vi "sv_Convert Units SRS.vi"(5 "desired units":i32(ring) items=["no change"=-1, "m/s^2"=0, "mm/s^2"=2, "micron/s^2"=3, "in/s^2"=1, "mil/s^2"=5], 6 "error in (no error)":errorcluster, 7 "channel info":T1={"sensor sensitivity"=1000.0, "engineering units"=1, "dB reference"=1.0, "custom label"="EU", "weighting filter"=0, "pregain"=0.0} {"pregain" format="%.2f"; "weighting filter" items=["Linear", "A-weighting", "B-weighting", "C-weighting", "ITU-R 468-4", "Dolby", "CCITT", "C-message", "Wb", "Wc", "Wd", "We", "Wf", "Wh", "Wj", "Wk", "Wm", "AES17 20 kHz lowpass", "AES17 40 kHz lowpass", "AES17 20 kHz highpass", "AES17 40 kHz highpass"]; "dB reference" format="%^.1e"; "engineering units" items=["custom..."=0, "V"=1, "A"=21, "C"=30, "pC"=31, "s"=32, "-"=29, "Pa"=2, "N"=20, "g"=3, "m/s^2"=4, "m/s"=5, "m"=6, "mm/s"=12, "mm"=13, "micron/s"=14, "micron"=15, "in/s^2"=7, "in/s"=8, "in"=9, "mil/s"=10, "mil"=11, "rad/s^2"=16, "rad/s"=17, "rad"=18, "deg/s^2"=26, "deg/s"=27, "deg"=28, "RPM"=22, "cycle/s^2"=23, "Hz"=24, "cycle"=25, "strain"=19]; "sensor sensitivity" format="%#_5f"}) -> (0 "error out":errorcluster, 1 "scale factor":dbl, 4 "unit label":string)   [LabVIEW 2017, in "SoundVib_Transient.lvlib"]
uses:
  <vilib>/addons/Sound and Vibration/svt_Transients/SoundVib_Transient.lvlib
  <vilib>/addons/_NISVFA/_Shared subVIs/Controls/svc_Channel Info.ctl
  <vilib>/addons/_NISVFA/_Shared subVIs/Controls/svc_Engineering Units Text Ring.ctl
  <vilib>/addons/_NISVFA/_Shared subVIs/Controls/svc_Weighting Filter Text Ring.ctl
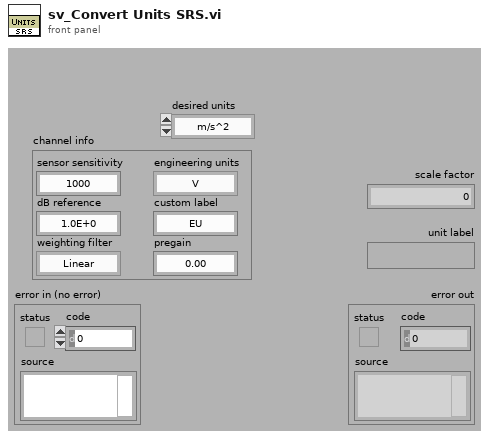
[diagram p1: front panel]
types:
  T1 = typedef "svc_Channel Info.ctl" = cluster{"sensor sensitivity":dbl, "engineering units":T2, "dB reference":dbl, "custom label":string, "weighting filter":T3, "pregain":dbl}
  T2 = typedef "svc_Engineering Units Text Ring.ctl" = u16
  T3 = typedef "svc_Weighting Filter Text Ring.ctl" = u16
  T4 = enum16{"custom...", "V", "Pa", "g", "m/s^2", "m/s", "m", "in/s^2", "in/s", "in", "mil/s", "mil", "mm/s", "mm", "micron/s", "micron", "rad/s^2", "rad/s", "rad", "strain", "N", "A", "rpm", "cycle/s^2", "Hz", "cycle", "deg/s^2", "deg/s", "deg", "Undefined", "C", "pC"}
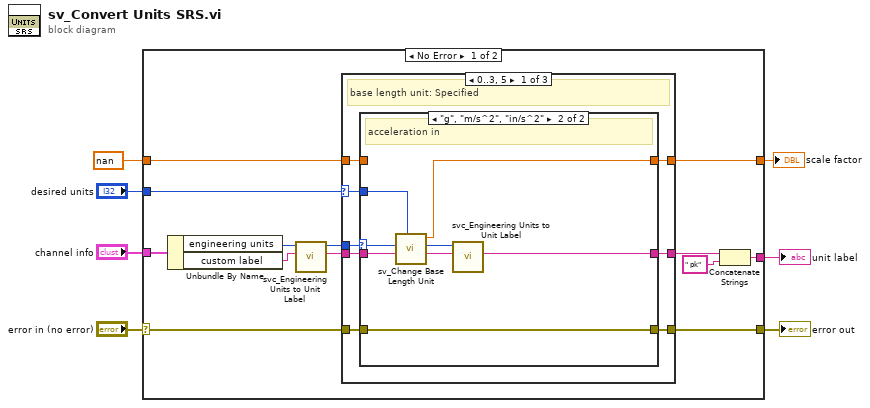
[diagram p0: block diagram]
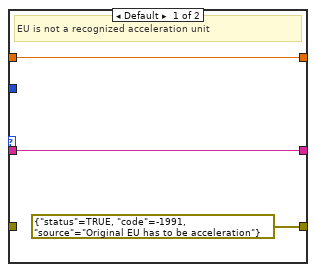
[diagram p2: hidden frame]
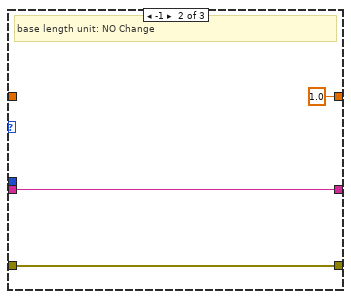
[diagram p3: hidden frame]
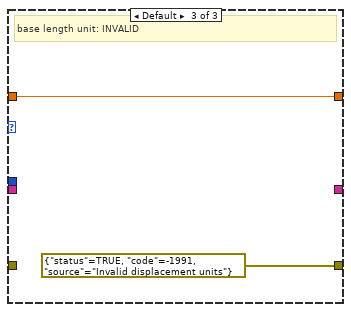
[diagram p4: hidden frame]
diagram:
  n1 = case shown="No Error" "error in (no error)" {
    selector: "error in (no error)" -> [w19 w46]
    tunnel: [w18 w46] -> w6
    tunnel: "channel info" -> [w20 _]
    tunnel: [w14 _] -> w4
    tunnel: "desired units" -> [w17 _]
    tunnel: [w13 w45] -> w2
    tunnel: nan ("value out [desired EU]") -> [w8 w45]
    frame No Error {
      n2 = Unbundle By Name(w20) -> ("engineering units"=w9:T2, "custom label"=w12:string)
      n3 = call <vilib>:"svc_Engineering Units to Unit Label.vi"("custom label"=w12, "engineering units"=w9) -> ("unit label"=w11:string, "engineering units enum"=w10:T4)  [unwired: 8 in]
      n4 = case shown="0..3, 5" w17 {
        selector: w17 -> [w24 _ _]
        tunnel: w11 -> [w27 w42 _]
        tunnel: w10 -> [w28 _ _]
        tunnel: [w26 w42 _] -> w15
        tunnel: [w25 w41 errorcluster {"status"=TRUE, "code"=-1991, "source"="Invalid displacement units"} ("error IO")] -> w18
        tunnel: w19 -> [w22 w41 _]
        tunnel: [w23 1.0 ("value out [desired EU]") w43] -> w13
        tunnel: w8 -> [w21 _ w43]
        frame 0..3, 5 {
          # "base length unit: Specified"
          n5 = case shown="\"g\", \"m/s^2\", \"in/s^2\"" w28 {
            selector: w28 -> [_ w35]
            tunnel: w27 -> [w30 w36]
            tunnel: [w30 w38] -> w26
            tunnel: [errorcluster {"status"=TRUE, "code"=-1991, "source"="Original EU has to be acceleration"} ("error IO") w37] -> w25
            tunnel: w24 -> [_ w39]
            tunnel: [w29 w34] -> w23
            tunnel: w22 -> [_ w37]
            tunnel: w21 -> [w29 _]
            frame Default {
              # "EU is not a recognized acceleration unit"
            }
            frame "g", "m/s^2", "in/s^2" {
              # "acceleration in"
              n6 = call <vilib>:"sv_Change Base Length Unit.vi"("desired base units for vibration"=w39, "custom label in"=w36, "engineering units in"=w35) -> ("custom label out"=w32:string, "engineering units out"=w33:T2, "value out [desired EU]"=w34:dbl)  [unwired: 4 in]
              n7 = call <vilib>:"svc_Engineering Units to Unit Label.vi"("custom label"=w32, "engineering units"=w33) -> ("unit label"=w38:string)  [unwired: 8 in, 1 out]
            }
          }
        }
        frame -1 {
          # "base length unit: NO Change"
        }
        frame Default {
          # "base length unit: INVALID"
        }
      }
      n8 = Concatenate Strings(w15, " pk" ("string")) -> (w14:string)
    }
    frame Error {
    }
  }
  "error out" <- w6
  "unit label" <- w4
  "scale factor" <- w2
